vi "ADI_IMU_ADIS16448_OffsetComp.vi"(1 "Yaw Axis":enum16{"X", "Y", "Z"}(ring)=enum."Z", 2 "Raw Data":dbl[](array[numeric])) -> (0 "Offset Compensated Data":dbl[](array[numeric]))   [LabVIEW 2018, in "ADIS16448_IMU.lvlib"]
uses:
  ADIS16448_IMU.lvlib
  <vilib>/ptbypt/NI_PtbyPt.lvlib
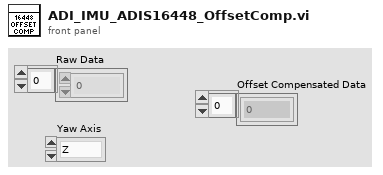
[diagram p1: front panel]
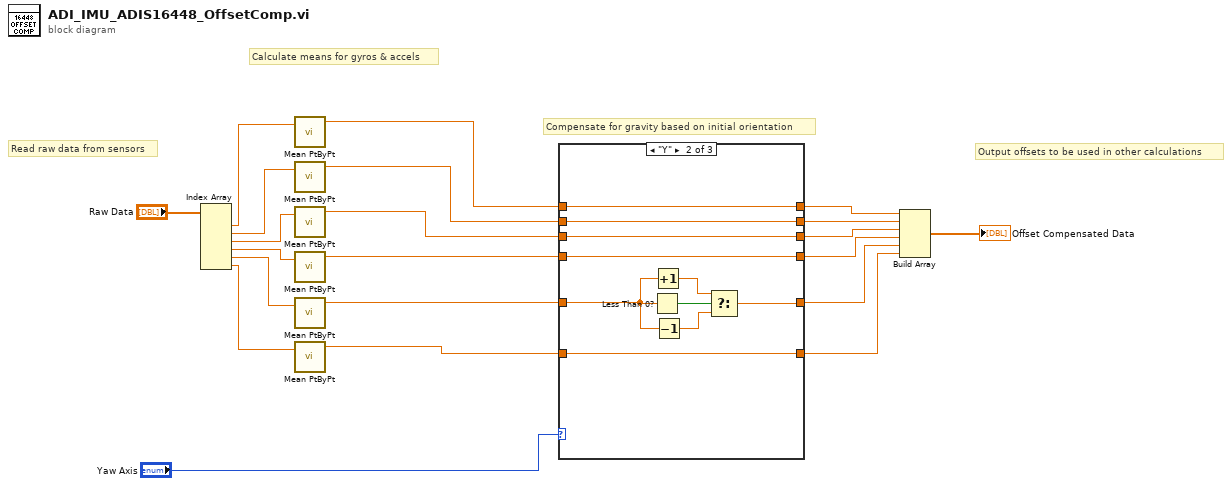
[diagram p0: block diagram]
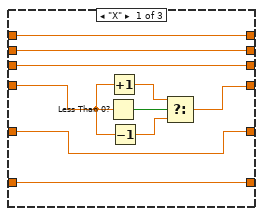
[diagram p2: hidden frame]
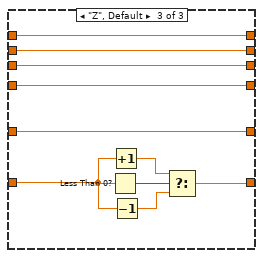
[diagram p3: hidden frame]
diagram:
  # "Output offsets to be used in other calculations"
  # "Compensate for gravity based on initial orientation"
  # "Calculate means for gyros & accels"
  # "Read raw data from sensors"
  n1 = Index Array(array="Raw Data") -> (element #1=w19:dbl, element #2=w20:dbl, element #3=w21:dbl, element #4=w18:dbl, element #5=w17:dbl, element #6=w16:dbl)  [unwired: 6 in]
  n2 = call <vilib>:"Mean PtByPt.vi"("x"=w19) -> ("mean"=w12:dbl)  [unwired: 3 in, 1 out]
  n3 = call <vilib>:"Mean PtByPt.vi"("x"=w20) -> ("mean"=w9:dbl)  [unwired: 3 in, 1 out]
  n4 = call <vilib>:"Mean PtByPt.vi"("x"=w21) -> ("mean"=w8:dbl)  [unwired: 3 in, 1 out]
  n5 = call <vilib>:"Mean PtByPt.vi"("x"=w18) -> ("mean"=w5:dbl)  [unwired: 3 in, 1 out]
  n6 = call <vilib>:"Mean PtByPt.vi"("x"=w17) -> ("mean"=w4:dbl)  [unwired: 3 in, 1 out]
  n7 = call <vilib>:"Mean PtByPt.vi"("x"=w16) -> ("mean"=w6:dbl)  [unwired: 3 in, 1 out]
  n8 = case shown="\"Y\"" "Yaw Axis" {
    tunnel: w12 -> [w31 w41 w51]
    tunnel: [w31 w41 w51] -> w11
    tunnel: [w30 w40 w50] -> w10
    tunnel: w9 -> [w30 w40 w50]
    tunnel: w8 -> [w29 w39 w49]
    tunnel: [w29 w39 w49] -> w7
    tunnel: w6 -> [w22 w32 w43]
    tunnel: [w25 w33 w48] -> w3
    tunnel: w5 -> [w24 w33 w48]
    tunnel: [w23 w35 w47] -> w2
    tunnel: w4 -> [w23 w34 w47]
    tunnel: [w22 w32 w46] -> w1
    frame "X" {
      n9 = Less Than 0?(x=w24) -> (x < 0?=w28:bool)
      n10 = Increment(x=w24) -> (x+1=w27:dbl)
      n11 = Decrement(x=w24) -> (x-1=w26:dbl)
      n12 = Select(t=w27, s=w28, f=w26) -> (s? t:f=w25:dbl)
    }
    frame "Y" {
      n13 = Less Than 0?(x=w34) -> (x < 0?=w38:bool)
      n14 = Increment(x=w34) -> (x+1=w37:dbl)
      n15 = Decrement(x=w34) -> (x-1=w36:dbl)
      n16 = Select(t=w37, s=w38, f=w36) -> (s? t:f=w35:dbl)
    }
    frame "Z", Default {
      n17 = Less Than 0?(x=w43) -> (x < 0?=w45:bool)
      n18 = Increment(x=w43) -> (x+1=w44:dbl)
      n19 = Decrement(x=w43) -> (x-1=w42:dbl)
      n20 = Select(t=w44, s=w45, f=w42) -> (s? t:f=w46:dbl)
    }
  }
  n21 = Build Array(w11, w10, w7, w3, w2, w1) -> (→"Offset Compensated Data":dbl[])
